vi "5-1.vi"() -> ()   [LabVIEW 2022 SP3, in "AoC22.lvlib"]
uses:
  AoC22.lvlib
  <vilib>/IlluminatedG/lv-stream/Stream.lvlib
panel:
  out "concatenated string":string
  out "Array 2":string[](array[string])
  out "Array":cluster{string[]}[](array[cluster])
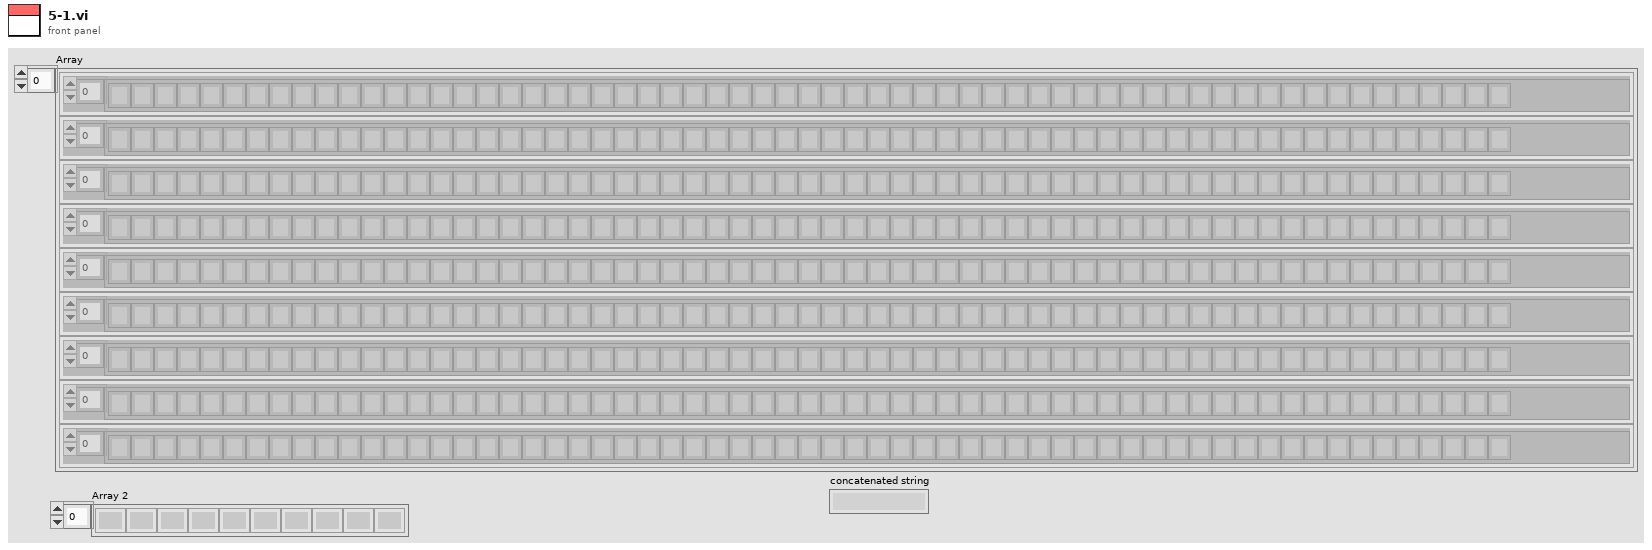
[diagram p1: front panel]
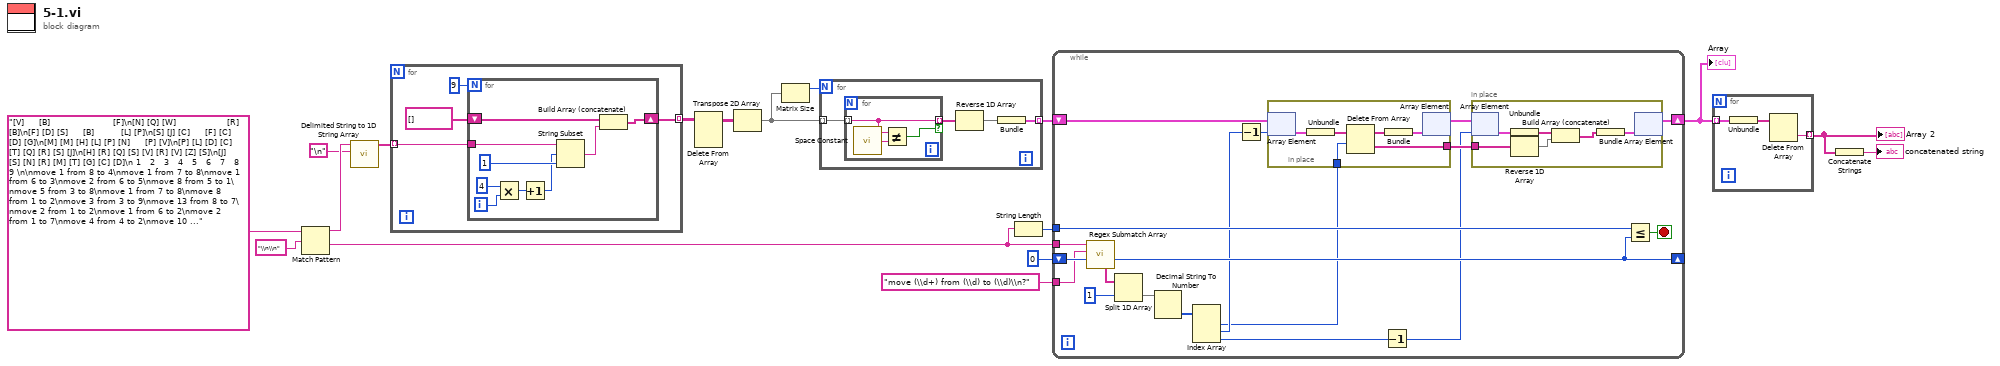
[diagram p0: block diagram]
diagram:
  n1 = Match Pattern(string="[V]     [B]                     [F]\n[N] [Q] [W]                 [R] [B]\n[F] [D] [S]     [B]         [L] [P]\n[S] [J] [C]     [F] [C]     [D] [G]\n[M] [M] [H] [L] [P] [N]     [P] [V]\n[P] [L] [D] [C] [T] [Q] [R] [S] [J]\n[H] [R] [Q] [S] [V] [R] [V] [Z] [S]\n[J] [S] [N] [R] [M] [T] [G] [C] [D]\n 1   2   3   4   5   6   7   8   9 \n\nmove 1 from 8 to 4\nmove 1 from 7 to 8\nmove 1 from 6 to 3\nmove 2 from 6 to 5\nmove 8 from 5 to 1\nmove 5 from 3 to 8\nmove 1 from 7 to 8\nmove 8 from 1 to 2\nmove 3 from 3 to 9\nmove 13 from 8 to 7\nmove 2 from 1 to 2\nmove 1 from 6 to 2\nmove 2 from 1 to 7\nmove 4 from 4 to 2\nmove 10 from 9 to 4\nmove 7 from 4 to 1\nmove 1 from 6 to 7\nmove 2 from 4 to 5\nmove 1 from 5 to 2\nmove 1 from 5 to 8\nmove 3 from 1 to 5\nmove 2 from 4 to 6\nmove 2 from 6 to 4\nmove 2 from 4 to 5\nmove 5 from 1 to 5\nmove 1 from 9 to 5\nmove 1 from 8 to 5\nmove 14 from 2 to 6\nmove 12 from 7 to 4\nmove 4 from 6 to 7\nmove 3 from 6 to 4\nmove 4 from 4 to 9\nmove 2 from 4 to 6\nmove 2 from 9 to 3\nmove 9 from 4 to 3\nmove 2 from 1 to 6\nmove 5 from 7 to 3\nmove 4 from 7 to 8\nmove 2 from 6 to 7\nmove 3 from 6 to 7\nmove 10 from 5 to 8\nmove 8 from 8 to 9\nmove 10 from 9 to 7\nmove 12 from 7 to 5\nmove 1 from 1 to 5\nmove 3 from 7 to 2\nmove 10 from 3 to 7\nmove 6 from 5 to 7\nmove 2 from 6 to 1\nmove 12 from 2 to 7\nmove 3 from 3 to 1\nmove 1 from 6 to 5\nmove 10 from 5 to 7\nmove 3 from 3 to 4\nmove 34 from 7 to 1\nmove 2 from 6 to 9\nmove 1 from 6 to 3\nmove 3 from 1 to 3\nmove 1 from 7 to 3\nmove 3 from 3 to 6\nmove 1 from 4 to 3\nmove 22 from 1 to 6\nmove 2 from 9 to 7\nmove 2 from 4 to 9\nmove 12 from 6 to 8\nmove 1 from 7 to 6\nmove 4 from 8 to 2\nmove 1 from 7 to 1\nmove 6 from 8 to 9\nmove 1 from 2 to 5\nmove 1 from 2 to 7\nmove 13 from 1 to 2\nmove 2 from 3 to 1\nmove 4 from 7 to 5\nmove 3 from 9 to 4\nmove 1 from 1 to 8\nmove 4 from 5 to 2\nmove 12 from 6 to 2\nmove 3 from 1 to 3\nmove 1 from 4 to 1\nmove 9 from 8 to 5\nmove 6 from 5 to 7\nmove 2 from 4 to 5\nmove 5 from 9 to 6\nmove 5 from 3 to 7\nmove 30 from 2 to 6\nmove 11 from 7 to 9\nmove 36 from 6 to 3\nmove 10 from 9 to 3\nmove 1 from 6 to 5\nmove 3 from 5 to 2\nmove 2 from 5 to 2\nmove 28 from 3 to 4\nmove 6 from 4 to 1\nmove 1 from 2 to 3\nmove 2 from 5 to 2\nmove 6 from 1 to 7\nmove 1 from 1 to 6\nmove 6 from 3 to 5\nmove 6 from 7 to 2\nmove 1 from 6 to 4\nmove 2 from 2 to 6\nmove 8 from 2 to 1\nmove 3 from 2 to 4\nmove 2 from 3 to 4\nmove 4 from 3 to 4\nmove 1 from 6 to 1\nmove 2 from 1 to 8\nmove 1 from 6 to 4\nmove 1 from 9 to 3\nmove 2 from 5 to 4\nmove 1 from 8 to 7\nmove 1 from 7 to 9\nmove 1 from 3 to 5\nmove 1 from 8 to 6\nmove 34 from 4 to 9\nmove 13 from 9 to 8\nmove 1 from 8 to 2\nmove 1 from 2 to 1\nmove 4 from 5 to 1\nmove 9 from 8 to 7\nmove 11 from 1 to 3\nmove 1 from 4 to 2\nmove 1 from 6 to 7\nmove 1 from 9 to 4\nmove 1 from 4 to 1\nmove 1 from 5 to 3\nmove 5 from 7 to 8\nmove 1 from 2 to 5\nmove 1 from 5 to 1\nmove 21 from 9 to 5\nmove 19 from 3 to 4\nmove 17 from 4 to 6\nmove 2 from 8 to 4\nmove 2 from 6 to 8\nmove 2 from 6 to 9\nmove 2 from 7 to 6\nmove 1 from 4 to 9\nmove 6 from 5 to 6\nmove 1 from 9 to 8\nmove 8 from 5 to 7\nmove 15 from 6 to 2\nmove 1 from 9 to 7\nmove 2 from 1 to 6\nmove 3 from 4 to 7\nmove 1 from 1 to 6\nmove 3 from 5 to 4\nmove 2 from 5 to 6\nmove 2 from 4 to 1\nmove 13 from 7 to 8\nmove 2 from 6 to 4\nmove 3 from 2 to 4\nmove 2 from 7 to 6\nmove 5 from 4 to 6\nmove 4 from 2 to 6\nmove 1 from 1 to 9\nmove 18 from 8 to 3\nmove 1 from 4 to 5\nmove 1 from 2 to 7\nmove 15 from 3 to 1\nmove 1 from 5 to 1\nmove 3 from 3 to 4\nmove 1 from 5 to 4\nmove 1 from 5 to 6\nmove 1 from 6 to 8\nmove 2 from 8 to 2\nmove 3 from 1 to 8\nmove 6 from 2 to 8\nmove 1 from 7 to 6\nmove 12 from 8 to 5\nmove 2 from 9 to 6\nmove 6 from 1 to 5\nmove 9 from 5 to 3\nmove 1 from 2 to 8\nmove 20 from 6 to 9\nmove 3 from 6 to 7\nmove 1 from 7 to 1\nmove 7 from 3 to 4\nmove 2 from 7 to 2\nmove 1 from 8 to 7\nmove 8 from 4 to 1\nmove 11 from 1 to 7\nmove 10 from 7 to 6\nmove 2 from 4 to 9\nmove 21 from 9 to 3\nmove 6 from 5 to 9\nmove 6 from 3 to 2\nmove 1 from 4 to 5\nmove 1 from 7 to 9\nmove 8 from 3 to 2\nmove 9 from 2 to 1\nmove 14 from 1 to 6\nmove 1 from 1 to 7\nmove 4 from 3 to 8\nmove 3 from 8 to 7\nmove 5 from 7 to 4\nmove 3 from 6 to 9\nmove 2 from 3 to 7\nmove 3 from 5 to 6\nmove 1 from 5 to 6\nmove 2 from 7 to 9\nmove 1 from 8 to 3\nmove 22 from 6 to 5\nmove 3 from 9 to 4\nmove 3 from 6 to 1\nmove 5 from 4 to 6\nmove 9 from 2 to 8\nmove 4 from 6 to 1\nmove 1 from 3 to 2\nmove 1 from 2 to 3\nmove 6 from 8 to 1\nmove 2 from 4 to 3\nmove 10 from 1 to 7\nmove 2 from 8 to 7\nmove 1 from 9 to 6\nmove 4 from 3 to 5\nmove 1 from 8 to 3\nmove 4 from 9 to 8\nmove 1 from 4 to 3\nmove 1 from 3 to 8\nmove 3 from 7 to 6\nmove 1 from 1 to 5\nmove 10 from 5 to 9\nmove 5 from 6 to 4\nmove 5 from 8 to 5\nmove 4 from 9 to 8\nmove 3 from 3 to 9\nmove 2 from 8 to 6\nmove 5 from 7 to 5\nmove 1 from 4 to 1\nmove 1 from 1 to 2\nmove 2 from 8 to 6\nmove 1 from 2 to 1\nmove 1 from 7 to 2\nmove 1 from 1 to 5\nmove 28 from 5 to 9\nmove 3 from 6 to 1\nmove 1 from 6 to 9\nmove 1 from 2 to 9\nmove 2 from 1 to 2\nmove 2 from 7 to 5\nmove 1 from 7 to 5\nmove 1 from 2 to 5\nmove 3 from 1 to 9\nmove 1 from 5 to 8\nmove 15 from 9 to 2\nmove 11 from 9 to 4\nmove 11 from 4 to 7\nmove 2 from 4 to 1\nmove 7 from 7 to 8\nmove 1 from 1 to 4\nmove 20 from 9 to 1\nmove 2 from 7 to 8\nmove 1 from 4 to 6\nmove 1 from 6 to 2\nmove 2 from 7 to 5\nmove 1 from 9 to 6\nmove 1 from 4 to 9\nmove 4 from 5 to 2\nmove 1 from 6 to 8\nmove 1 from 4 to 9\nmove 11 from 8 to 3\nmove 1 from 1 to 9\nmove 1 from 5 to 9\nmove 1 from 2 to 6\nmove 4 from 9 to 8\nmove 4 from 8 to 7\nmove 10 from 1 to 6\nmove 7 from 1 to 5\nmove 8 from 3 to 4\nmove 2 from 3 to 5\nmove 3 from 7 to 4\nmove 1 from 4 to 5\nmove 2 from 1 to 6\nmove 9 from 2 to 6\nmove 1 from 7 to 9\nmove 1 from 3 to 2\nmove 7 from 4 to 3\nmove 3 from 3 to 7\nmove 5 from 2 to 3\nmove 1 from 1 to 9\nmove 2 from 2 to 7\nmove 1 from 4 to 6\nmove 3 from 5 to 6\nmove 4 from 7 to 6\nmove 1 from 7 to 4\nmove 1 from 4 to 7\nmove 1 from 2 to 8\nmove 1 from 7 to 1\nmove 27 from 6 to 2\nmove 1 from 4 to 1\nmove 7 from 5 to 7\nmove 1 from 4 to 1\nmove 1 from 8 to 3\nmove 3 from 7 to 3\nmove 2 from 1 to 6\nmove 2 from 9 to 1\nmove 18 from 2 to 1\nmove 2 from 7 to 5\nmove 12 from 3 to 4\nmove 1 from 5 to 6\nmove 3 from 6 to 1\nmove 24 from 1 to 8\nmove 9 from 2 to 4\nmove 3 from 2 to 1\nmove 2 from 6 to 3\nmove 1 from 6 to 9\nmove 1 from 5 to 6\nmove 1 from 6 to 2\nmove 1 from 1 to 7\nmove 1 from 2 to 1\nmove 1 from 1 to 2\nmove 3 from 7 to 2\nmove 2 from 1 to 4\nmove 8 from 4 to 5\nmove 22 from 8 to 1\nmove 1 from 8 to 1\nmove 13 from 4 to 1\nmove 1 from 8 to 5\nmove 3 from 3 to 1\nmove 1 from 2 to 7\nmove 38 from 1 to 6\nmove 27 from 6 to 1\nmove 2 from 2 to 9\nmove 3 from 9 to 8\nmove 2 from 8 to 6\nmove 1 from 8 to 3\nmove 1 from 2 to 1\nmove 1 from 3 to 6\nmove 1 from 2 to 3\nmove 1 from 7 to 6\nmove 7 from 6 to 3\nmove 20 from 1 to 4\nmove 6 from 1 to 6\nmove 17 from 4 to 7\nmove 3 from 6 to 5\nmove 14 from 7 to 9\nmove 8 from 5 to 7\nmove 3 from 1 to 6\nmove 3 from 3 to 1\nmove 2 from 4 to 1\nmove 4 from 5 to 1\nmove 9 from 6 to 2\nmove 3 from 6 to 4\nmove 4 from 7 to 8\nmove 4 from 1 to 6\nmove 2 from 3 to 1\nmove 6 from 6 to 7\nmove 4 from 8 to 7\nmove 4 from 2 to 1\nmove 4 from 2 to 3\nmove 4 from 9 to 5\nmove 8 from 9 to 5\nmove 1 from 9 to 5\nmove 1 from 2 to 1\nmove 16 from 7 to 2\nmove 10 from 2 to 9\nmove 11 from 9 to 8\nmove 4 from 3 to 5\nmove 3 from 1 to 4\nmove 13 from 5 to 7\nmove 10 from 8 to 5\nmove 2 from 1 to 5\nmove 11 from 7 to 4\nmove 2 from 3 to 6\nmove 3 from 7 to 6\nmove 1 from 3 to 2\nmove 1 from 1 to 8\nmove 2 from 8 to 4\nmove 3 from 1 to 2\nmove 4 from 6 to 1\nmove 7 from 1 to 9\nmove 1 from 6 to 7\nmove 2 from 5 to 8\nmove 1 from 2 to 9\nmove 1 from 7 to 8\nmove 5 from 5 to 8\nmove 1 from 2 to 3\nmove 4 from 2 to 5\nmove 17 from 4 to 1\nmove 10 from 5 to 9\nmove 2 from 4 to 2\nmove 2 from 4 to 1\nmove 1 from 4 to 9\nmove 1 from 3 to 7\nmove 1 from 7 to 8\nmove 12 from 9 to 2\nmove 1 from 2 to 4\nmove 1 from 4 to 1\nmove 1 from 1 to 9\nmove 1 from 8 to 1\nmove 8 from 8 to 3\nmove 2 from 5 to 1\nmove 3 from 1 to 9\nmove 1 from 2 to 6\nmove 4 from 3 to 7\nmove 1 from 7 to 6\nmove 10 from 9 to 2\nmove 1 from 5 to 9\nmove 1 from 9 to 3\nmove 17 from 1 to 6\nmove 2 from 1 to 2\nmove 11 from 6 to 7\nmove 2 from 2 to 9\nmove 2 from 9 to 5\nmove 12 from 7 to 9\nmove 20 from 2 to 7\nmove 5 from 9 to 5\nmove 21 from 7 to 1\nmove 2 from 6 to 4\nmove 11 from 1 to 4\nmove 5 from 4 to 6\nmove 1 from 7 to 8\nmove 5 from 9 to 3\nmove 5 from 2 to 8\nmove 3 from 9 to 3\nmove 2 from 8 to 7\nmove 2 from 1 to 7\nmove 10 from 6 to 3\nmove 1 from 2 to 6\nmove 2 from 8 to 5\nmove 1 from 6 to 5\nmove 2 from 4 to 9\nmove 1 from 4 to 5\nmove 8 from 1 to 6\nmove 4 from 4 to 8\nmove 6 from 8 to 4\nmove 21 from 3 to 9\nmove 5 from 9 to 2\nmove 4 from 7 to 9\nmove 22 from 9 to 3\nmove 9 from 6 to 4\nmove 2 from 2 to 6\nmove 2 from 2 to 1\nmove 2 from 5 to 7\nmove 7 from 5 to 4\nmove 22 from 4 to 2\nmove 2 from 5 to 4\nmove 16 from 2 to 5\nmove 2 from 6 to 2\nmove 13 from 3 to 4\nmove 5 from 5 to 7\nmove 15 from 4 to 7\nmove 3 from 2 to 3\nmove 3 from 2 to 5\nmove 1 from 1 to 2\nmove 1 from 2 to 4\nmove 6 from 5 to 9\nmove 4 from 3 to 6\nmove 2 from 5 to 9\nmove 1 from 2 to 7\nmove 1 from 1 to 9\nmove 2 from 4 to 5\nmove 19 from 7 to 8\nmove 1 from 6 to 5\nmove 1 from 5 to 1\nmove 1 from 9 to 4\nmove 5 from 8 to 1\nmove 3 from 8 to 1\nmove 7 from 5 to 6\nmove 3 from 7 to 1\nmove 1 from 2 to 5\nmove 4 from 9 to 8\nmove 2 from 5 to 6\nmove 10 from 1 to 4\nmove 1 from 7 to 2\nmove 6 from 3 to 4\nmove 9 from 4 to 3\nmove 2 from 2 to 8\nmove 2 from 9 to 5\nmove 5 from 8 to 3\nmove 1 from 1 to 5\nmove 2 from 5 to 6\nmove 1 from 1 to 7\nmove 2 from 9 to 7\nmove 8 from 4 to 7\nmove 3 from 3 to 9\nmove 4 from 6 to 3\nmove 1 from 5 to 3\nmove 1 from 7 to 2\nmove 1 from 2 to 1\nmove 1 from 6 to 5\nmove 1 from 5 to 2\nmove 10 from 7 to 4\nmove 10 from 4 to 1\nmove 10 from 1 to 8\nmove 1 from 9 to 6\nmove 1 from 1 to 4\nmove 11 from 8 to 1\nmove 2 from 9 to 5\nmove 5 from 6 to 3\nmove 1 from 3 to 8\nmove 4 from 1 to 3\nmove 5 from 3 to 8\nmove 1 from 4 to 7\nmove 1 from 7 to 2\nmove 13 from 3 to 5\nmove 2 from 2 to 1\nmove 4 from 3 to 1\nmove 4 from 5 to 6\nmove 3 from 6 to 2\nmove 4 from 5 to 4\nmove 8 from 8 to 7\nmove 1 from 3 to 9", regular expression="\\n\\n") -> (before substring=w15:string, after substring=w5:string)  [unwired: 1 in, 2 out]
  n2 = call <vilib>:"Delimited String to 1D String Array.vi"("delimiter"="\n", "delimited string"=w15) -> ("string array"=w13:string[])  [unwired: 9 in]
  n3 = for {
    tunnel: w13 -> [w20] mode=indexing
    tunnel: [w18] -> w12 mode=indexing
    n4 = for {
      N: 9 -> [_]
      tunnel: w20 -> [w30]
      shift-right: [w23] -> w18
      shift-left: string[] [] -> [w24]
      i -> [w27]
      n5 = Multiply(x=4, y=w27) -> (x*y=w28:i32)
      n6 = Increment(x=w28) -> (x+1=w25:i32)
      n7 = String Subset(string=w30, offset (0)=w25, length (rest)=1 ("length (rest)")) -> (substring=w22:string)
      n8 = Build Array (concatenate)(w24, w22) -> (w23:string[])
    }
  }
  n9 = Delete From Array(array=w12) -> (array with subset deleted=w11:string[][])  [unwired: 3 in, 1 out]
  n10 = Transpose 2D Array(2D array=w11) -> (transposed array=w9:string[][])
  n11 = Matrix Size(0:w9) -> (1:w10:i32)  [unwired: 1 out]
  n12 = for {
    N: w10 -> [_]
    tunnel: w9 -> [w34] mode=indexing
    tunnel: [w32] -> w8 mode=indexing
    n13 = for {
      tunnel: w34 -> [w36] mode=indexing
      tunnel: [w36] -> w33 mode=indexing if=w35
      n14 = call <vilib>:"Space Constant.vi"() -> ("String"=w37:string)
      n15 = Not Equal?(x=w36, y=w37) -> (x != y?=w35:bool)
    }
    n16 = Reverse 1D Array(array=w33) -> (reversed array=w31:string[])
    n17 = Bundle(w31) -> (w32:cluster{string[]})  [unwired: 1 in]
  }
  n18 = String Length(string=w5) -> (length=w4:i32)
  n19 = while {
    shift-right: [w41] -> w3
    shift-left: w8 -> [w40]
    tunnel: w5 -> [w56]
    shift-right: [w52] -> _
    shift-left: 0 -> [w55]
    tunnel: "move (\\d+) from (\\d) to (\\d)\\n?" -> [w54]
    tunnel: w4 -> [w53]
    stop <- w51 stop-if-true
    n20 = call <vilib>:"Regex Submatch Array.vi"("offset (0)"=w55, "regular expression"=w54, "string"=w56) -> ("offset past match"=w52:i32, "matches"=w50:string[])  [unwired: 6 in, 1 out]
    n21 = Split 1D Array(array=w50, index=1) -> (second subarray=w48:string[])  [unwired: 1 out]
    n22 = Decimal String To Number(string=w48) -> (number=w47:i32[])  [unwired: 2 in, 1 out]
    n23 = Index Array(array=w47) -> (element #1=w45:i32, element #2=w46:i32, element #3=w43:i32)  [unwired: 3 in]
    n24 = Decrement(x=w46) -> (x-1=w39:i32)
    n25 = in-place {
      in-place-border: w45 -> [w66]
      in-place-border: [w63] -> w42
      n26 = in-place-array #1(w40, w39) -> (w68:cluster{string[]})
      n27 = Unbundle(w68) -> (w67:string[])
      n28 = Delete From Array(array=w67, length=w66) -> (deleted portion=w63:string[], array with subset deleted=w65:string[])  [unwired: 1 in]
      n29 = Bundle(w65) -> (w64:cluster{string[]})  [unwired: 1 in]
      n30 = in-place-array #1(w64) -> (w44:cluster{string[]}[])  [unwired: 1 out]
    }
    n31 = Decrement(x=w43) -> (x-1=w38:i32)
    n32 = in-place {
      in-place-border: w42 -> [w58]
      n33 = in-place-array #2(w44, w38) -> (w62:cluster{string[]})
      n34 = Unbundle(w62) -> (w60:string[])
      n35 = Reverse 1D Array(array=w58) -> (reversed array=w57:string[])
      n36 = Build Array (concatenate)(w60, w57) -> (w59:string[])
      n37 = Bundle(w59) -> (w61:cluster{string[]})  [unwired: 1 in]
      n38 = in-place-array #2(w61) -> (w41:cluster{string[]}[])  [unwired: 1 out]
    }
    n39 = Less Or Equal?(x=w53, y=w52) -> (x <= y?=w51:bool)
  }
  "Array" <- w3
  n40 = for {
    tunnel: w3 -> [w71] mode=indexing
    tunnel: [w69] -> w2 mode=indexing
    n41 = Unbundle(w71) -> (w70:string[])
    n42 = Delete From Array(array=w70) -> (deleted portion=w69:string)  [unwired: 2 in, 1 out]
  }
  "Array 2" <- w2
  n43 = Concatenate Strings(w2) -> (→"concatenated string":string)
